vi "Configure Syringe.vi"(7 "Config Manager":refnum<class "Config Manager Class.lvclass">, 8 "error in":errorcluster, 11 "WorkTable in":refnum<class "WorkTable Class.lvclass">) -> (0 "error out":errorcluster, 3 "WorkTable out":refnum<class "WorkTable Class.lvclass">)   [LabVIEW 2017, in "WorkTable Class.lvclass"]
uses:
  WorkTable Class.lvclass
  Type Definitions/Worktable_Syringe.ctl
  Vec3d Class/Vec3d Class.lvclass
  Config Manager Class/Config Manager Class.lvclass
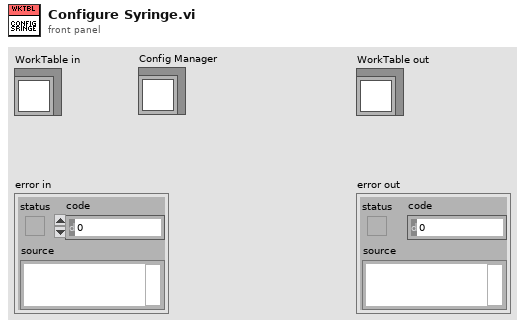
[diagram p1: front panel]
types:
  T1 = typedef "Worktable_Syringe.ctl" = cluster{"Syringe Holder":string, "Mixing Time":timestamp, "Tip Offset":refnum<class "Vec3d Class.lvclass">}
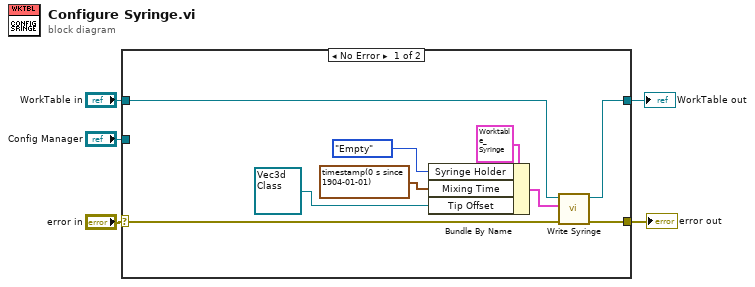
[diagram p0: block diagram]
diagram:
  n1 = case shown="No Error" "error in" {
    selector: "error in" -> [w7 w16]
    tunnel: "WorkTable in" -> [w13 w15]
    tunnel: [w11 w16] -> w3
    tunnel: [w14 w15] -> w2
    tunnel: "Config Manager" -> [_ _]
    frame No Error {
      n2 = Bundle By Name(cluster=T1 {"Syringe Holder"="", "Mixing Time"=timestamp(0 s since 1904-01-01), "Tip Offset"=refnum} ("Syringe"), "Syringe Holder"=enum16{"Empty", "Populated", "Calibrated"}."Empty", "Mixing Time"=timestamp(0 s since 1904-01-01), "Tip Offset"=refnum<class "Vec3d Class.lvclass"> refnum) -> (w8:T1)
      n3 = call-dynamic "Write Syringe.vi"("error in (no error)"=w7, "Syringe"=w8, "WorkTable Class in"=w13) -> ("error out"=w11:errorcluster, "WorkTable Class out"=w14:refnum<class "WorkTable Class.lvclass">)  [unwired: 7 in]
    }
    frame Error {
    }
  }
  "WorkTable out" <- w2
  "error out" <- w3
